vi "Find Speeds and Angles.vi"(5 "Prev Angles":dbl[](array[numeric]), 6 "Gyro Angle":dbl, 7 "Twist Axis":dbl, 8 "Y Axis":dbl, 9 "X Axis":dbl) -> (0 "Speeds":dbl[](array[numeric]), 3 "Angles":dbl[](array[numeric]))   [LabVIEW 2020]
doc: "Performs all calculations necessary for the implementation of Swerve Drive.\n\n X Axis:\nThe X Axis of Driving Joystick (Strafing). Range: [-1, 1].\n Y Axis:\nThe X Axis of Driving Joystick (Strafing). Range: [-1, 1].\n Twist Axis:\nThe Twist Axis of Driving Joystick (Twist). Range: [-1, 1].\n Gyro:\nAngle of Gyro 0. Range: [0, 360].\n Previous Angles:\nList of angles of each wheel as measured by the absolute encode. Ranges [0, 360]"
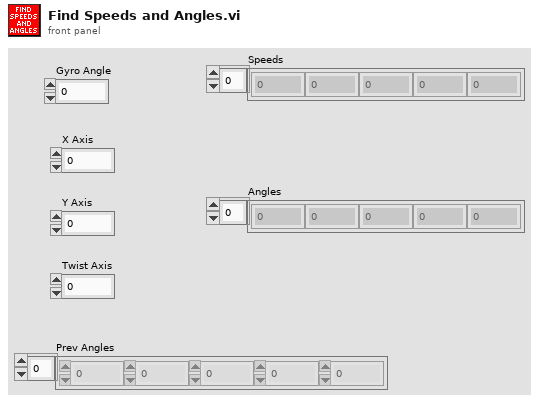
[diagram p1: front panel]
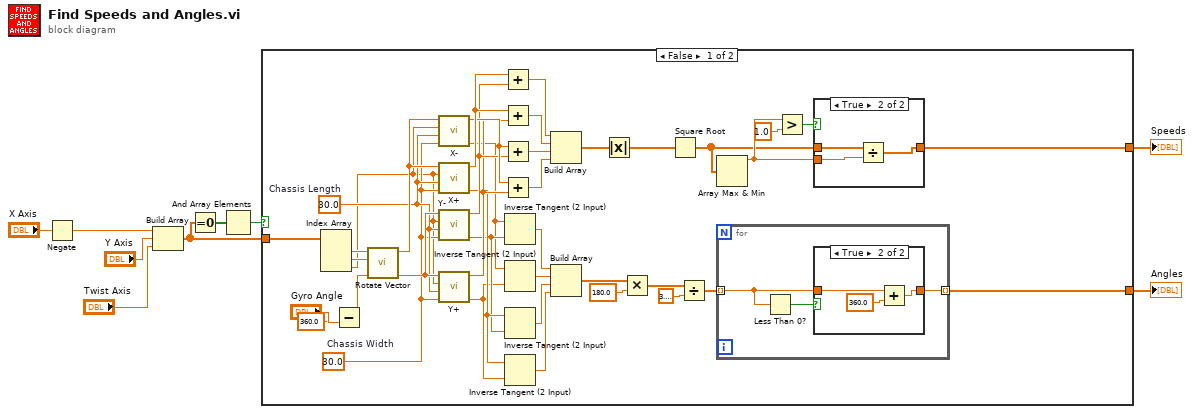
[diagram p0: block diagram]
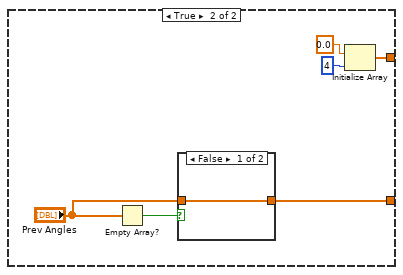
[diagram p4: hidden frame]
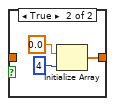
[diagram p5: hidden frame]
diagram:
  n1 = Negate(x="X Axis") -> (-x=w2:dbl)
  n2 = Build Array(w2, "Y Axis", "Twist Axis") -> (w8:dbl[])
  n3 = Equal To 0?(x=w8) -> (x = 0?=w7:bool[])
  n4 = And Array Elements(Boolean array=w7) -> (logical AND=w6:bool)
  n5 = case shown="False" w6 {
    tunnel: w8 -> [w18 _]
    tunnel: [w14 w61] -> w5
    tunnel: [w13 w65] -> w4
    frame False {
      w23 = 30.0  # Chassis Width
      w24 = 30.0  # Chassis Length
      n6 = Index Array(array=w18) -> (element #1=w17:dbl, element #2=w16:dbl, element #3=w15:dbl)  [unwired: 3 in]
      n7 = Subtract(x=360.0, y="Gyro Angle") -> (x-y=w12:dbl)
      n8 = call "Rotate Vector.vi"("Angle"=w12, "Y"=w16, "X"=w17) -> ("Y'"=w25:dbl, "X'"=w26:dbl)  [unwired: 7 in]
      n9 = call "X-.vi"("Width"=w23, "Length"=w24, "Z"=w15, "X"=w26) -> ("X-"=w42:dbl, "(X-)^2"=w47:dbl)  [unwired: 6 in]
      n10 = call "X+.vi"("Width"=w23, "Length"=w24, "Z"=w15, "X"=w26) -> ("X+"=w44:dbl, "(X+)^2"=w48:dbl)  [unwired: 6 in]
      n11 = call "Y-.vi"("Width"=w23, "Length"=w24, "Z"=w15, "Y"=w25) -> ("Y-"=w43:dbl, "(Y-)^2"=w46:dbl)  [unwired: 6 in]
      n12 = call "Y+.vi"("Width"=w23, "Length"=w24, "Z"=w15, "Y"=w25) -> ("Y+"=w41:dbl, "(Y+)^2"=w45:dbl)  [unwired: 6 in]
      n13 = Add(x=w48, y=w46) -> (x+y=w22:dbl)
      n14 = Add(x=w48, y=w45) -> (x+y=w21:dbl)
      n15 = Add(x=w47, y=w46) -> (x+y=w20:dbl)
      n16 = Add(x=w47, y=w45) -> (x+y=w19:dbl)
      n17 = Inverse Tangent (2 Input)(1:w43, 2:w42) -> (0:w37:dbl)
      n18 = Inverse Tangent (2 Input)(1:w41, 2:w42) -> (0:w36:dbl)
      n19 = Inverse Tangent (2 Input)(1:w43, 2:w44) -> (0:w35:dbl)
      n20 = Inverse Tangent (2 Input)(1:w41, 2:w44) -> (0:w34:dbl)
      n21 = Build Array(w22, w21, w20, w19) -> (w40:dbl[])
      n22 = Build Array(w37, w36, w35, w34) -> (w33:dbl[])
      n23 = Absolute Value(x=w40) -> (abs(x)=w28:dbl[])
      n24 = Multiply(x=w33, y=180.0) -> (x*y=w31:dbl[])
      n25 = Square Root(x=w28) -> (sqrt(x)=w27:dbl[])
      n26 = Divide(x=w31, y=3.141592653589793) -> (x/y=w29:dbl[])
      n27 = Array Max & Min(array=w27) -> (max value=w39:dbl)  [unwired: 3 out]
      n28 = for {
        tunnel: w29 -> [w51] mode=indexing
        tunnel: [w50] -> w13 mode=indexing
        n29 = Less Than 0?(x=w51) -> (x < 0?=w52:bool)
        n30 = case shown="True" w52 {
          tunnel: w51 -> [w53 w56]
          tunnel: [w53 w54] -> w50
          frame False {
          }
          frame True {
            n31 = Add(x=w56, y=360.0) -> (x+y=w54:dbl)
          }
        }
      }
      n32 = Greater?(x=w39, y=1.0) -> (0:w38:bool)
      n33 = case shown="True" w38 {
        tunnel: w27 -> [w57 w60]
        tunnel: w39 -> [_ w58]
        tunnel: [w57 w59] -> w14
        frame False {
        }
        frame True {
          n34 = Divide(x=w60, y=w58) -> (x/y=w59:dbl[])
        }
      }
    }
    frame True {
      n35 = Empty Array?(array="Prev Angles") -> (empty?=w66:bool)
      n36 = case shown="False" w66 {
        tunnel: [w67 w70] -> w65
        tunnel: "Prev Angles" -> [w67 _]
        frame False {
        }
        frame True {
          n37 = Initialize Array(0.0 ("element"), 4 ("dimension size")) -> (w70:dbl[])
        }
      }
      n38 = Initialize Array(0.0 ("element"), 4 ("dimension size")) -> (w61:dbl[])
    }
  }
  "Speeds" <- w5
  "Angles" <- w4
